vi "load_hardware_from_enum.vi"(8 "error in (no error)":errorcluster, 11 "hardware type":T1) -> (0 "error out":errorcluster, 3 "Hardware out":refnum<class "Hardware.lvclass">)   [LabVIEW 2017, in "Hardware.lvclass"]
doc: "Load the hardware from an hardware enum"
uses:
  Hardware.lvclass
  hardware_type.ctl
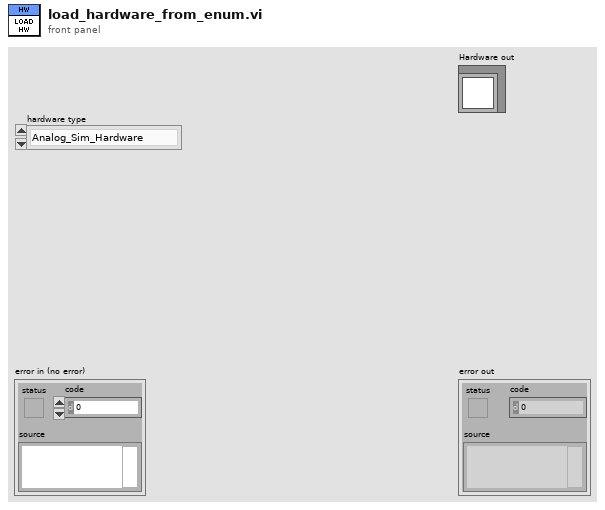
[diagram p1: front panel]
types:
  T1 = typedef "Hardware.lvclass/hardware_type.ctl" = enum16{"Analog_Sim_Hardware", "Digital_Sim_Hardware", "AI_Ni_Hardware", "AO_Ni_Hardware", "DI_Ni_Hardware", "DO_Ni_Hardware"}
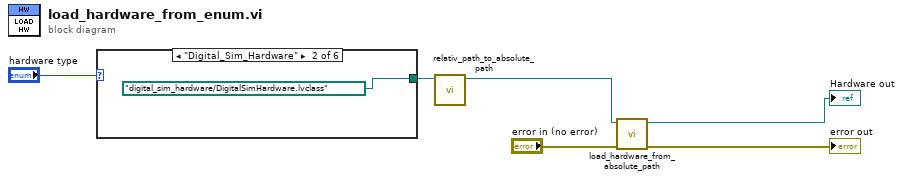
[diagram p0: block diagram]
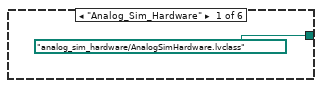
[diagram p2: hidden frame]
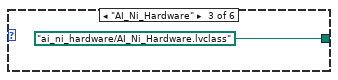
[diagram p3: hidden frame]
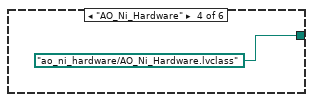
[diagram p4: hidden frame]
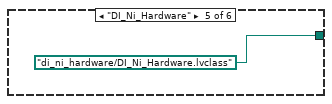
[diagram p5: hidden frame]
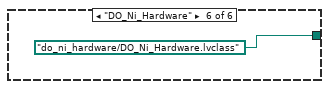
[diagram p6: hidden frame]
diagram:
  n1 = case shown="\"Digital_Sim_Hardware\"" "hardware type" {
    tunnel: [path "analog_sim_hardware/AnalogSimHardware.lvclass" path "digital_sim_hardware/DigitalSimHardware.lvclass" path "ai_ni_hardware/AI_Ni_Hardware.lvclass" path "ao_ni_hardware/AO_Ni_Hardware.lvclass" path "di_ni_hardware/DI_Ni_Hardware.lvclass" path "do_ni_hardware/DO_Ni_Hardware.lvclass"] -> w5
    frame "Analog_Sim_Hardware" {
    }
    frame "Digital_Sim_Hardware" {
    }
    frame "AI_Ni_Hardware" {
    }
    frame "AO_Ni_Hardware" {
    }
    frame "DI_Ni_Hardware" {
    }
    frame "DO_Ni_Hardware" {
    }
  }
  n2 = call "relativ_path_to_absolute_path.vi"("relativ path"=w5) -> ("absolute path"=w4:path)  [unwired: 10 in]
  n3 = call "load_hardware_from_absolute_path.vi"("error in (no error)"="error in (no error)", "absolute path"=w4) -> ("error out"=→"error out":errorcluster, "Hardware out"=→"Hardware out":refnum<class "Hardware.lvclass">)  [unwired: 8 in]
